vi "Pre Launch Init.vi"(11 "Cobra RT in":refnum<class "Cobra RT.lvclass">) -> (0 "error out":errorcluster, 3 "Cobra RT out":refnum<class "Cobra RT.lvclass">)   [LabVIEW 2019, in "Cobra RT.lvlib" / "Cobra RT.lvclass"]
doc: "(<B>Filename</B>: Actor Framework.lvlib:Actor.lvclass:Pre Launch Init.vi)\n\nDefines behavior that occurs after the Launch Nested Actor method is invoked but before the actor's Actor Core method begins running.\n\nBy default, this method does nothing. A descendant class may override it to define behavior."
uses:
  Cobra RT.lvclass
  Cobra RT.lvclass/Cobra RT.ctl
  <vilib>/MGI/Panel Manager/Panel Actor/Panel Actor/Panel Actor.lvclass
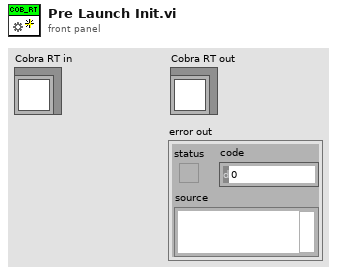
[diagram p1: front panel]
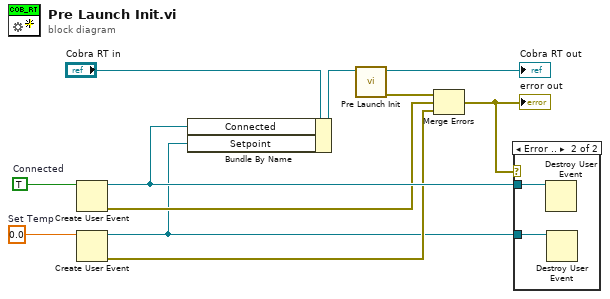
[diagram p0: block diagram]
diagram:
  w2 = 0.0  # Set Temp
  w10 = TRUE  # Connected
  n1 = Create User Event(user event datatype=w10) -> (user event=w7:refnum<user-event>, error out=w5:errorcluster)  [unwired: 1 in]
  n2 = Create User Event(user event datatype=w2) -> (user event=w1:refnum<user-event>, error out=w4:errorcluster)  [unwired: 1 in]
  n3 = Bundle By Name(cluster="Cobra RT in", "Connected"=w7, "Setpoint"=w1) -> (w8:refnum<class "Cobra RT.lvclass">)
  n4 = call-parent "Pre Launch Init.vi"("Panel Actor in"=w8) -> ("error out"=w6:errorcluster, "Panel Actor out"=→"Cobra RT out":refnum<class "Cobra RT.lvclass">)  [unwired: 9 in]
  n5 = Merge Errors(w6, w5, w4) -> (w3:errorcluster)
  "error out" <- w3
  n6 = case shown="Error .." w3 {
    tunnel: w7 -> [_ w13]
    tunnel: w1 -> [_ w12]
    frame No Error {
    }
    frame Error {
      n7 = Destroy User Event(user event=w13) -> ()  [unwired: 1 in, 1 out]
      n8 = Destroy User Event(user event=w12) -> ()  [unwired: 1 in, 1 out]
    }
  }
